vi "Wrapper.vi"(0 "Update Device Configuration in":refnum<class "Update Device Configuration MSG.lvclass">, 1 "CVT Session":T1, 5 "error in":errorcluster) -> (19 "error out":errorcluster)   [LabVIEW 2014, in "Controller.lvlib" / "Update Device Configuration MSG.lvclass"]
uses:
  Update Device Configuration MSG.lvclass
  <userlib>/_Session Fwk/Typedefs/Session Handle.ctl
  <userlib>/_Session Fwk/Session - Root.lvclass
  Device Configuration/Get Serialized Device Configuration MSG.lvclass/Get Serialized Device Configuration MSG.ctl
  Device Configuration/Read cfg cluster.vi
  reusable/Session APIs/CVT/CVT.lvclass
panel:
  out "SerializedString":string
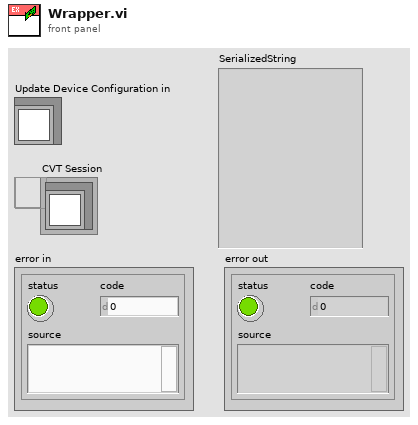
[diagram p1: front panel]
types:
  T1 = typedef "Session - Root.lvclass/Session Handle.ctl" = refnum<data-value>
  T2 = typedef "Cfg Msg.ctl" = cluster{"ID":string, "type":string, "label":string, "SN":string, "controller_":bool, "Addr":string, "Model":string}
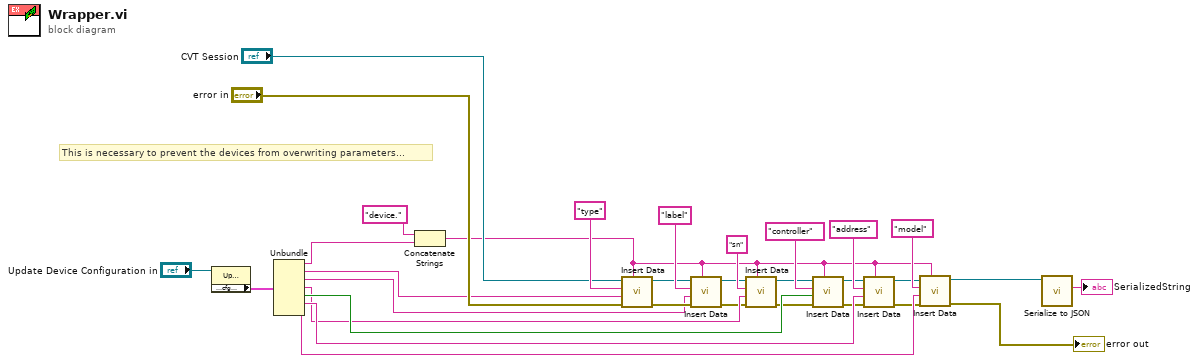
[diagram p0: block diagram]
diagram:
  # "This is necessary to prevent the devices from overwriting parameters..."
  n1 = property class="Update Device Configuration"(reference="Update Device Configuration in") -> ("Accessors:cfg cluster"=w7:T2)  [unwired: 1 in, 2 out]
  n2 = Unbundle(w7) -> ("ID"=w5:string, "type"=w10:string, "label"=w12:string, "SN"=w17:string, "controller_"=w21:bool, "Addr"=w24:string, "Model"=w29:string)
  n3 = Concatenate Strings("device." ("string"), w5) -> (w3:string)
  n4 = call "Insert Data.vi"("Group"=w3, "error in"="error in", "Data"=w10, "tag"="type", "CVT Session In"="CVT Session") -> ("error out"=w31:errorcluster, "CVT Session Out"=w11:T1)  [unwired: 5 in]
  n5 = call "Insert Data.vi"("Group"=w3, "error in"=w31, "Data"=w12, "tag"="label", "CVT Session In"=w11) -> ("error out"=w15:errorcluster, "CVT Session Out"=w14:T1)  [unwired: 5 in]
  n6 = call "Insert Data.vi"("Group"=w3, "error in"=w15, "Data"=w17, "tag"="sn", "CVT Session In"=w14) -> ("error out"=w19:errorcluster, "CVT Session Out"=w18:T1)  [unwired: 5 in]
  n7 = call "Insert Data.vi"("Group"=w3, "error in"=w19, "Data"=w21, "tag"="controller", "CVT Session In"=w18) -> ("error out"=w23:errorcluster, "CVT Session Out"=w22:T1)  [unwired: 5 in]
  n8 = call "Insert Data.vi"("Group"=w3, "error in"=w23, "Data"=w24, "tag"="address", "CVT Session In"=w22) -> ("error out"=w26:errorcluster, "CVT Session Out"=w27:T1)  [unwired: 5 in]
  n9 = call "Insert Data.vi"("Group"=w3, "error in"=w26, "Data"=w29, "tag"="model", "CVT Session In"=w27) -> ("error out"=→"error out":errorcluster, "CVT Session Out"=w2:T1)  [unwired: 5 in]
  n10 = call "Serialize to JSON.vi"("CVT Session In"=w2) -> ("SerializedString"=→"SerializedString":string)  [unwired: 8 in, 2 out]
